vi "Transceiver Thread.Transfer.Build.vi"(8 "error in (no error)":errorcluster, 10 "Transfer":refnum<class "Transfer.lvclass">, 11 "Transceiver Thread in":refnum<class "Transceiver Thread.lvclass">) -> (0 "error out":errorcluster, 3 "Transceiver Thread out":refnum<class "Transceiver Thread.lvclass">)   [LabVIEW 2017, in "DSF.Engine.lvlib" / "Transceiver Thread.lvclass"]
uses:
  Transceiver Thread.lvclass
  Transfer/Transfer.lvclass
  Transfer/Transfer.lvclass/Transfer.ctl
  Transceiver Thread.lvclass/Transceiver Thread.ctl
  Pointer/DBL Pointer.lvclass/DBL Pointer.ctl
  <vilib>/NI/Memory Manager/Classes/Pointer/Memory.Pointer.lvclass/Memory.Pointer.ctl
  Pointer/DBL Pointer.Get Channel Count.vi
  <vilib>/NI/Memory Manager/Classes/Pointer/Memory.Pointer.Read.vi
  <vilib>/NI/Memory Manager/Classes/Pointer/Memory.Pointer.Read.1D.DBL.vi
  <vilib>/NI/Memory Manager/Classes/Pointer/Memory.Pointer.Read.No Check.1D.DBL.vi
  <vilib>/NI/Memory Manager/Classes/Pointer/Memory.Pointer.Parameter Check.Null Pointer.vi
  <vilib>/NI/Memory Manager/Classes/Pointer/Memory.Pointer.Parameter Check.Subset.Power of 2.vi
  <vilib>/NI/Memory Manager/Classes/Pointer/Memory.Pointer.Get Address.vi
  <vilib>/NI/Memory Manager/Classes/Pointer/Memory.Pointer.Errors.vi
  <vilib>/NI/Memory Manager/Classes/Pointer/Memory.Pointer.Errors.Null Pointer.vi
  <vilib>/NI/Memory Manager/Classes/Pointer/Memory.Pointer.Errors.Out of Bounds.vi
  <vilib>/NI/Memory Manager/Classes/Pointer/Memory.Pointer.Get Size.vi
  <vilib>/NI/Memory Manager/Classes/Pointer/Memory.Pointer.Count to Size.Power of 2.vi
  <vilib>/NI/Memory Manager/Classes/Pointer/Memory.Pointer.Errors.Create Error.vi
  <vilib>/NI/Memory Manager/VIs/Source.Write.String.vi
  <vilib>/NI/Memory Manager/Classes/Pointer/Memory.Pointer.Errors.Write Pointer Size.vi
  <vilib>/NI/Memory Manager/VIs/Source.Write.Scalar.Base10.vi
  <vilib>/NI/Memory Manager/VIs/Source.Write.Scalar.Base10 (U64).vi
  <vilib>/NI/Memory Manager/VIs/New Error Cluster Constant.vi
  <vilib>/NI/Memory Manager/VIs/New Error Cluster Constant (512B).vi
  <vilib>/NI/Memory Manager/VIs/Error Cluster.Set Status.vi
  <vilib>/NI/Memory Manager/VIs/Error Cluster.Set Code.vi
  <vilib>/NI/Memory Manager/VIs/Error Cluster.Set VI Source.vi
  <vilib>/NI/Memory Manager/Constants/Memory.Constants.vi
  <vilib>/NI/Memory Manager/Constants/Memory.Constants.Library Name.vi
  <vilib>/NI/Memory Manager/Classes/Pointer/Memory.Pointer.Errors.Get Info.vi
  Pointer/DBL Pointer.lvclass
  C:/Program Files (x86)/National Instruments/LabVIEW 2017/vi.lib/NI/Memory Manager/Classes/Pointer/Memory.Pointer.lvclass
  Buffer/Buffer.Write.vi
  Buffer/Buffer.Write.1D.U64.vi
  Buffer/Buffer.Write.1D.U32.vi
  Buffer/Buffer.Write.1D.U16.vi
  Buffer/Buffer.Write.1D.U8.vi
  Buffer/Buffer.Write.1D.I64.vi
  Buffer/Buffer.Write.1D.I32.vi
  Buffer/Buffer.Write.1D.I16.vi
  Buffer/Buffer.Write.1D.I8.vi
  Buffer/Buffer.Write.1D.DBL.vi
  Buffer/Buffer.Write.1D.SGL.vi
  Buffer/Buffer.Write.1D.Bool.vi
  Buffer/Buffer.lvclass
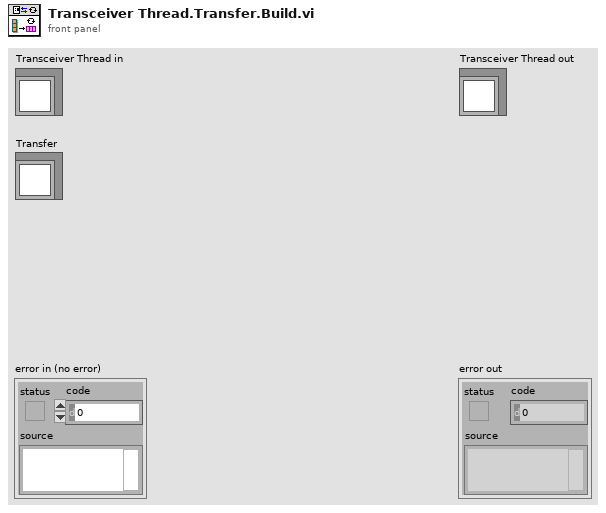
[diagram p1: front panel]
types:
  T1 = typedef "DSF.Engine.lvlib/DSF Runtime Channel Block.ctl" = cluster{"data type":T2, "count":u64, "buffer offset":u64}
  T2 = typedef "DSF Configuration API.lvlib/DSF Data Type.ctl" = enum8{"Bool", "SGL", "DBL", "I8", "I16", "I32", "I64", "U8", "U16", "U32", "U64"}
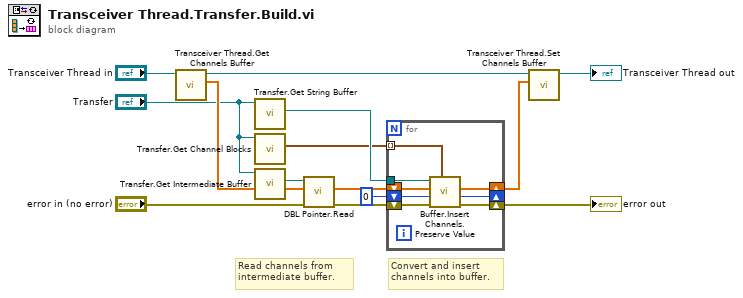
[diagram p0: block diagram]
diagram:
  # "Convert and insert channels into buffer."
  # "Read channels from intermediate buffer."
  n1 = call "Transceiver Thread.Get Channels Buffer.vi"("Transceiver Thread in"="Transceiver Thread in") -> ("channels buffer"=w7:dbl[], "Transceiver Thread out"=w5:refnum<class "Transceiver Thread.lvclass">)  [unwired: 9 in]
  n2 = call "Transfer.Get String Buffer.vi"("Transfer in"="Transfer") -> ("Buffer"=w13:refnum<class "Buffer.lvclass">)  [unwired: 9 in, 1 out]
  n3 = call "Transfer.Get Channel Blocks.vi"("Transfer in"="Transfer") -> ("channel blocks"=w2:T1[])  [unwired: 9 in, 1 out]
  n4 = call "Transfer.Get Intermediate Buffer.vi"("Transfer in"="Transfer") -> ("DBL Buffer"=w12:refnum<class "DBL Pointer.lvclass">)  [unwired: 9 in, 1 out]
  n5 = call "DBL Pointer.Read.vi"("error in (no error)"="error in (no error)", "buffer in"=w7, "DBL Pointer in"=w12) -> ("error out"=w9:errorcluster, "buffer out"=w10:dbl[])  [unwired: 6 in, 1 out]
  n6 = for {
    shift-right: [w20] -> w6
    shift-left: w10 -> [w21]
    shift-right: [w19] -> w14
    shift-left: w9 -> [w22]
    tunnel: w13 -> [w18]
    tunnel: w2 -> [w17] mode=indexing
    shift-right: [w16] -> _
    shift-left: u64 0 ("channels buffer index in") -> [w15]
    n7 = call "Buffer.Insert Channels.Preserve Value.vi"("channel block"=w17, "error in (no error)"=w22, "channels buffer index in"=w15, "channels buffer in"=w21, "Buffer in"=w18) -> ("error out"=w19:errorcluster, "channels buffer index out"=w16:u64, "channels buffer out"=w20:dbl[])  [unwired: 3 in, 1 out]
  }
  "error out" <- w14
  n8 = call "Transceiver Thread.Set Channels Buffer.vi"("channels buffer"=w6, "Transceiver Thread in"=w5) -> ("Transceiver Thread out"=→"Transceiver Thread out":refnum<class "Transceiver Thread.lvclass">)  [unwired: 9 in]
